vi "Write TSP Net Remote Instrument Data.vi"(6 "String":string, 7 "Command":string, 8 "error in (no error)":errorcluster, 9 "Data Type (0: String)":i32(ring) items=["String", "Command"], 10 "Instrument ID":string, 11 "VISA resource name":refnum<visa-resource-name>) -> (0 "error out":errorcluster, 3 "VISA resource name out":refnum<visa-resource-name>)   [LabVIEW 2020, in "Keithley 2600 Series.lvlib"]
doc: "Writes data to the remote instrument."
uses:
  <instrlib>/Keithley 2600 Series/Keithley 2600 Series.lvlib
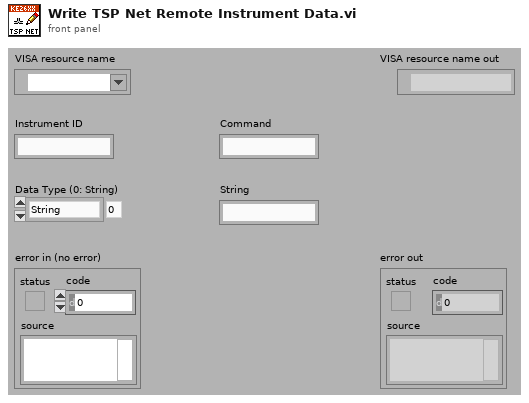
[diagram p1: front panel]
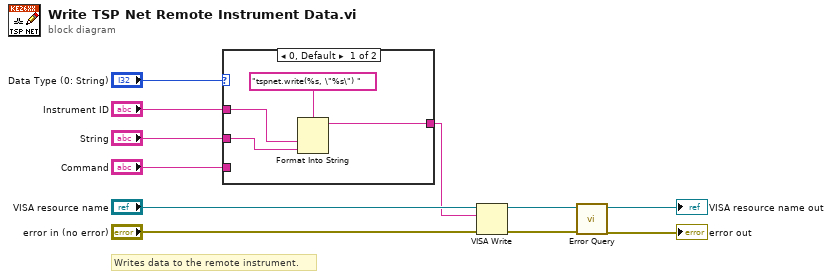
[diagram p0: block diagram]
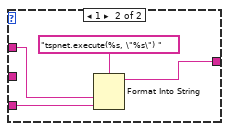
[diagram p2: hidden frame]
diagram:
  # "Writes data to the remote instrument."
  n1 = case shown="0, Default" "Data Type (0: String)" {
    tunnel: "Command" -> [_ w18]
    tunnel: "Instrument ID" -> [w13 w17]
    tunnel: [w12 w16] -> w2
    tunnel: "String" -> [w14 _]
    frame 0, Default {
      n2 = Format Into String(format string="tspnet.write(%s, \"%s\") ", w13, w14) -> (resulting string=w12:string)  [unwired: 2 in, 1 out]
    }
    frame 1 {
      n3 = Format Into String(format string="tspnet.execute(%s, \"%s\") ", w17, w18) -> (resulting string=w16:string)  [unwired: 2 in, 1 out]
    }
  }
  n4 = VISA Write(VISA resource name="VISA resource name", write buffer=w2, error in (no error)="error in (no error)") -> (VISA resource name out=w9:refnum<visa-resource-name>, error out=w8:errorcluster)  [unwired: 1 out]
  n5 = call <instrlib>:"Error Query.vi"("error in (no error)"=w8, "VISA resource name"=w9) -> ("error out"=→"error out":errorcluster, "VISA resource name out"=→"VISA resource name out":refnum<visa-resource-name>)  [unwired: 6 in, 2 out]
